vi "KeyDown.vi"(6 "PlatMods":T9, 7 "Type":T1, 8 "error in (no error)":errorcluster, 9 "VKey":T10, 10 "Char":i16, 11 "Data in":T2={"Class"={"Ants"=refnum, "Layer"=refnum, "Templates"=refnum, "Icon"=refnum, "Glyph"=refnum, "Settings"=refnum, "Tools"=refnum}, "Ref"={"Add Layer"=refnum, "Remove Layer"=refnum, "Line Text"=[], "Body Text Spec"=refnum, "DNL_Font"=refnum, "glyph path str"=refnum, "templates path str"=refnum, "Arrow Up"=refnum, "Arrow Down"=refnum, "IE VI Ref"=refnum, "Glyphs tree"=refnum, "Templates tree"=refnum, "Layer Icon Text"=refnum, "Layer Template"=refnum, "Clipboard"=refnum, "BW icon in"=refnum, "Color icon in"=refnum, "Layer Clust"=refnum, "Body Text"=refnum, "DNL_Framework Templates"=refnum, "Search Templates"=refnum, "TextMarker"=refnum, "Tab Control"=refnum, "Search Glyphs"=refnum, "Line Color"=refnum, "DNL_Glyphs []"=refnum, "Fill Color"=refnum, "Tools"=refnum, "Glyphs tree"=refnum, "Icon"=refnum, "Preview"=refnum, "Ants"=refnum, "Terminals"=refnum, "menu reference"=refnum, "LayerNames"=[], "GlyphLoadAnimation"=refnum, "TemplateLoadAnimation"=refnum, "refreshGlyphs"=refnum, "refreshTemplates"=refnum}, "Support"={"AntsRect"={"left"=0, "top"=0, "right"=0, "bottom"=0}, "Mouse Move Coords"={"Horizontal"=0, "Vertical"=0}, "Mouse Down Coords"={"Horizontal"=0, "Vertical"=0}, "Temp Coord"={"Horizontal"=0, "Vertical"=0}, "Action"=enum."Default", "Edge Color"=4914962, "Fill Color"=16860, "Mouse Down?"=FALSE, "Draft Mode?"=FALSE, "Temp Icon"=bytes[3102], "CTRL Pressed"=FALSE, "Move Selection?"=FALSE, "AntsRect Orig"={"left"=0, "top"=0, "right"=0, "bottom"=0}, "Text"="", "TM Set?"=FALSE, "Mouse inside icon?"=FALSE, "Tool (old value)"=0, "Pencil Move Color"=0, "Swap Colors?"=FALSE, "Shift pressed?"=FALSE}}) -> (0 "error out":errorcluster, 1 "Discard?":bool, 3 "Data out":T2={"Class"={"Ants"=refnum, "Layer"=refnum, "Templates"=refnum, "Icon"=refnum, "Glyph"=refnum, "Settings"=refnum, "Tools"=refnum}, "Ref"={"Add Layer"=refnum, "Remove Layer"=refnum, "Line Text"=[], "Body Text Spec"=refnum, "DNL_Font"=refnum, "glyph path str"=refnum, "templates path str"=refnum, "Arrow Up"=refnum, "Arrow Down"=refnum, "IE VI Ref"=refnum, "Glyphs tree"=refnum, "Templates tree"=refnum, "Layer Icon Text"=refnum, "Layer Template"=refnum, "Clipboard"=refnum, "BW icon in"=refnum, "Color icon in"=refnum, "Layer Clust"=refnum, "Body Text"=refnum, "DNL_Framework Templates"=refnum, "Search Templates"=refnum, "TextMarker"=refnum, "Tab Control"=refnum, "Search Glyphs"=refnum, "Line Color"=refnum, "DNL_Glyphs []"=refnum, "Fill Color"=refnum, "Tools"=refnum, "Glyphs tree"=refnum, "Icon"=refnum, "Preview"=refnum, "Ants"=refnum, "Terminals"=refnum, "menu reference"=refnum, "LayerNames"=[], "GlyphLoadAnimation"=refnum, "TemplateLoadAnimation"=refnum, "refreshGlyphs"=refnum, "refreshTemplates"=refnum}, "Support"={"AntsRect"={"left"=0, "top"=0, "right"=0, "bottom"=0}, "Mouse Move Coords"={"Horizontal"=0, "Vertical"=0}, "Mouse Down Coords"={"Horizontal"=0, "Vertical"=0}, "Temp Coord"={"Horizontal"=0, "Vertical"=0}, "Action"=enum."Default", "Edge Color"=4914962, "Fill Color"=16860, "Mouse Down?"=FALSE, "Draft Mode?"=FALSE, "Temp Icon"=bytes[3102], "CTRL Pressed"=FALSE, "Move Selection?"=FALSE, "AntsRect Orig"={"left"=0, "top"=0, "right"=0, "bottom"=0}, "Text"="", "TM Set?"=FALSE, "Mouse inside icon?"=FALSE, "Tool (old value)"=0, "Pencil Move Color"=0, "Swap Colors?"=FALSE, "Shift pressed?"=FALSE}})   [LabVIEW 2021]
uses:
  <vilib>/event_ctls.llb/eventvkey.ctl
  Controls/IE Data.ctl
  Class/Ants/Ants.lvclass
  Class/FakedArray/FakedArray.lvclass
  vi.lib/LabVIEW Icon API/lv_icon/Classes/Icon/Icon.lvclass
  Class/Icon Library/Glyph.lvclass
  Class/Settings/Settings.lvclass
  Class/Tools/Tools Paint.lvclass
  Controls/IE Classes.ctl
  Controls/References Cluster.ctl
  Controls/SupportClass.ctl
  <vilib>/Utility/miscctls.llb/LVPoint32TypeDef.ctl
  Controls/SupportClass_Action.ctl
  vi.lib/LabVIEW Icon API/lv_icon/Controls/IEColor.ctl
  <vilib>/event_ctls.llb/lveventtype.ctl
  vi.lib/LabVIEW Icon API/lv_icon/lv_icon.lvlib
panel:
  in  "Layer name":string="Clipboard"
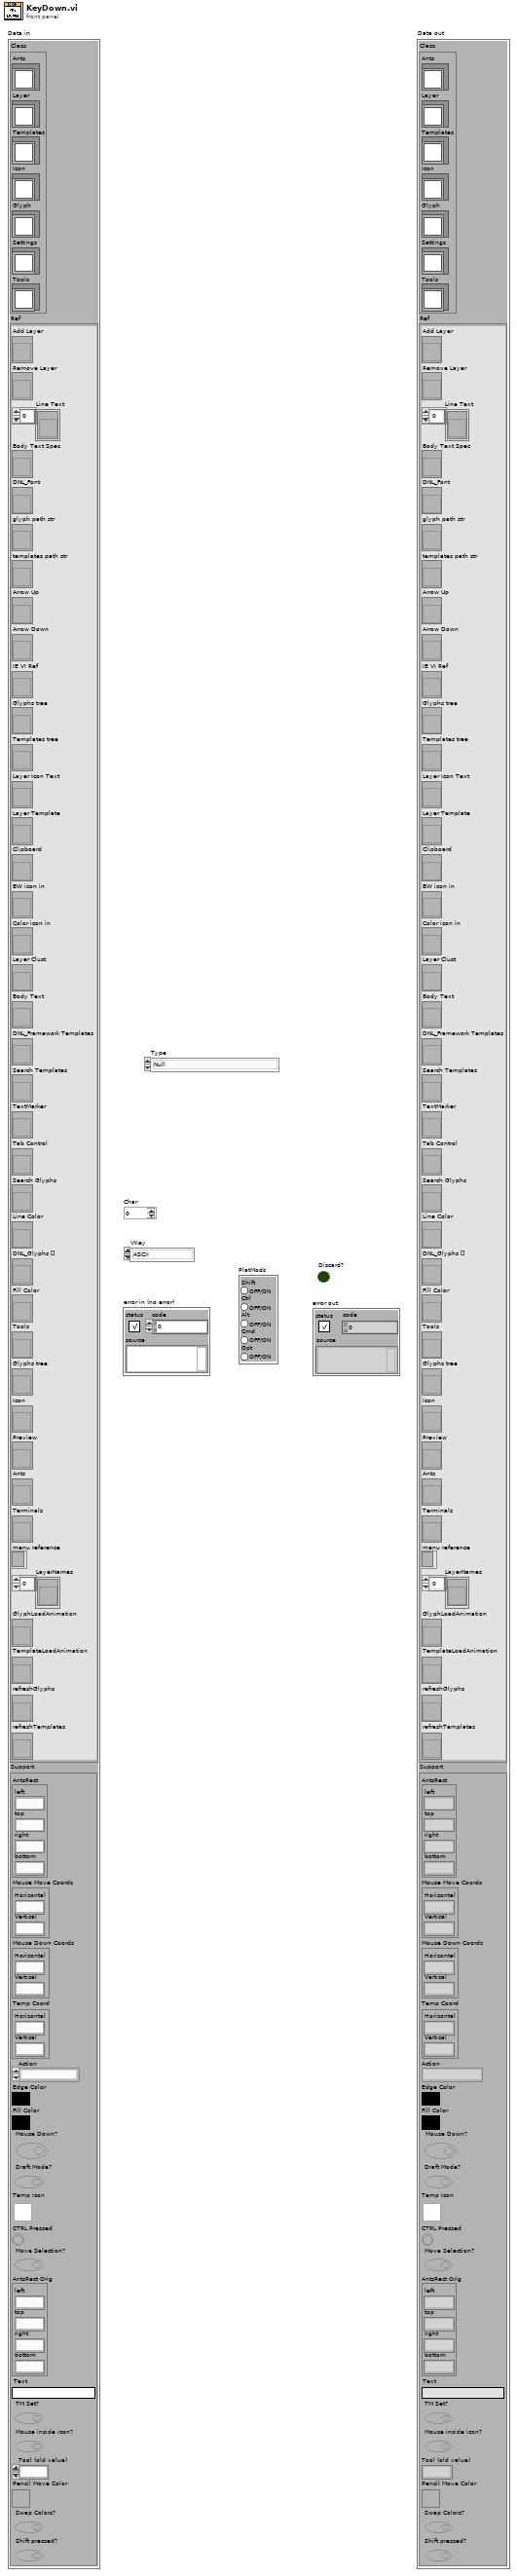
[diagram p1: front panel]
types:
  T1 = typedef "lveventtype.ctl" = enum32{"Null", "Timeout", "Annotation Menu Selection", "Annotation Menu Selection?", "App Instance Close", "App Instance Close?", "Autoscale Range Change", "Bookmark Info Change", "Cell Edit", "Cell Edit?", "Cursor Grab", "Cursor Grab?", "Cursor Menu Selection", "Cursor Menu Selection?", "Cursor Move", "Cursor Release", "Data Change", "Direction Change", "Display State Change", "Drag Ended", "Drag Enter", "Drag Leave", "Drag Over", "Drag Source Update", "Drag Starting", "Drag Starting?", "Drop", "Exec State Change", "Key Down", "Key Down?", "Key Repeat", "Key Repeat?", "Key Up", "Listbox Double Click", "Menu Activation?", "Menu Selection (App)", "Menu Selection? (App)", "Menu Selection (User)", "Mouse Down", "Mouse Down?", "Mouse Enter", "Mouse Leave", "Mouse Move", "Mouse Up", "Mouse Wheel", "NI Security User Change (App)", "Pane Size", "Panel Close", "Panel Close?", "Panel Resize", "Plot Attribute Change", "Scale Range Change", "Shortcut Menu Activation?", "Shortcut Menu Selection (App)", "Shortcut Menu Selection? (App)", "Shortcut Menu Selection (User)", "Tree Double Click", "Tree Drag", "Tree Drag?", "Tree Drop", "Tree Drop?", "Tree Item Close", "Tree Item Close?", "Tree Item Open", "Tree Item Open?", "User Event", "Value Change"}
  T2 = typedef "IE Data.ctl" = cluster{"Class":T3, "Ref":T4, "Support":T5}
  T3 = typedef "IE Classes.ctl" = cluster{"Ants":refnum<class "Ants.lvclass">, "Layer":refnum<class "FakedArray.lvclass">, "Templates":refnum<class "FakedArray.lvclass">, "Icon":refnum<class "Icon.lvclass">, "Glyph":refnum<class "Glyph.lvclass">, "Settings":refnum<class "Settings.lvclass">, "Tools":refnum<class "Tools Paint.lvclass">}
  T4 = typedef "References Cluster.ctl" = cluster{"Add Layer":refnum<vi>, "Remove Layer":refnum<vi>, "Line Text":refnum<vi>[], "Body Text Spec":refnum<vi>, "DNL_Font":refnum<vi>, "glyph path str":refnum<vi>, "templates path str":refnum<vi>, "Arrow Up":refnum<vi>, "Arrow Down":refnum<vi>, "IE VI Ref":refnum<vi>, "Glyphs tree":refnum<vi>, "Templates tree":refnum<vi>, "Layer Icon Text":refnum<vi>, "Layer Template":refnum<vi>, "Clipboard":refnum<vi>, "BW icon in":refnum<vi>, "Color icon in":refnum<vi>, "Layer Clust":refnum<vi>, "Body Text":refnum<vi>, "DNL_Framework Templates":refnum<vi>, "Search Templates":refnum<vi>, "TextMarker":refnum<vi>, "Tab Control":refnum<vi>, "Search Glyphs":refnum<vi>, "Line Color":refnum<vi>, "DNL_Glyphs []":refnum<vi>, "Fill Color":refnum<vi>, "Tools":refnum<vi>, "Glyphs tree":refnum<vi>, "Icon":refnum<vi>, "Preview":refnum<vi>, "Ants":refnum<vi>, "Terminals":refnum<vi>, "menu reference":refnum<k9>, "LayerNames":refnum<vi>[], "GlyphLoadAnimation":refnum<vi>, "TemplateLoadAnimation":refnum<vi>, "refreshGlyphs":refnum<vi>, "refreshTemplates":refnum<vi>}
  T5 = typedef "SupportClass.ctl" = cluster{"AntsRect":cluster{"left":i16, "top":i16, "right":i16, "bottom":i16}, "Mouse Move Coords":T6, "Mouse Down Coords":T6, "Temp Coord":T6, "Action":T7, "Edge Color":T8, "Fill Color":T8, "Mouse Down?":bool, "Draft Mode?":bool, "Temp Icon":picture, "CTRL Pressed":bool, "Move Selection?":bool, "AntsRect Orig":cluster{"left":i16, "top":i16, "right":i16, "bottom":i16}, "Text":string, "TM Set?":bool, "Mouse inside icon?":bool, "Tool (old value)":u32, "Pencil Move Color":u32, "Swap Colors?":bool, "Shift pressed?":bool}
  T6 = typedef "LVPoint32TypeDef.ctl" = cluster{"Horizontal":i32, "Vertical":i32}
  T7 = typedef "SupportClass_Action.ctl" = enum16{"Default", "Move Selection", "Glyph Library", "Tool"}
  T8 = typedef "IEColor.ctl" = u32
  T9 = cluster{"Shift":bool, "Ctrl":bool, "Alt":bool, "Cmd":bool, "Opt":bool}
  T10 = typedef "eventvkey.ctl" = enum16{"ASCII", "Enter", "Return", "Shift", "Ctrl", "Alt", "Cmd", "Opt", "Caps", "NumLock", "Clear", "Break", "Up", "Down", "Left", "Right", "Insert", "Delete", "Home", "End", "PageUp", "PageDown", "Escape", "Help", "Pause", "ScrollLock", "F1", "F2", "F3", "F4", "F5", "F6", "F7", "F8", "F9", "F10", "F11", "F12", "F13", "F14", "F15", "F16", "F17", "F18", "F19", "F20", "F21", "F22", "F23", "F24", "Play", "VolumeUp", "VolumeDown", "Mute", "Two Byte Char"}
  T11 = cluster{"left":i16, "top":i16, "right":i16, "bottom":i16}
  T12 = enum32{"Pencil", "Line", "Dropper", "Fill", "Rectangle", "Filled Rectangle", "Ellipse", "Filled Ellipse", "Eraser", "Text", "Select", "Move"}
  T13 = typedef "Graphic.ctl" = cluster{"Rectangle":cluster{"left":i16, "top":i16, "right":i16, "bottom":i16}, "Path":path, "Image":picture, "Filter":string, "FileName":string}
  T14 = cluster{"left":i16, "top":i16, "bottom":i16, "right":i16}
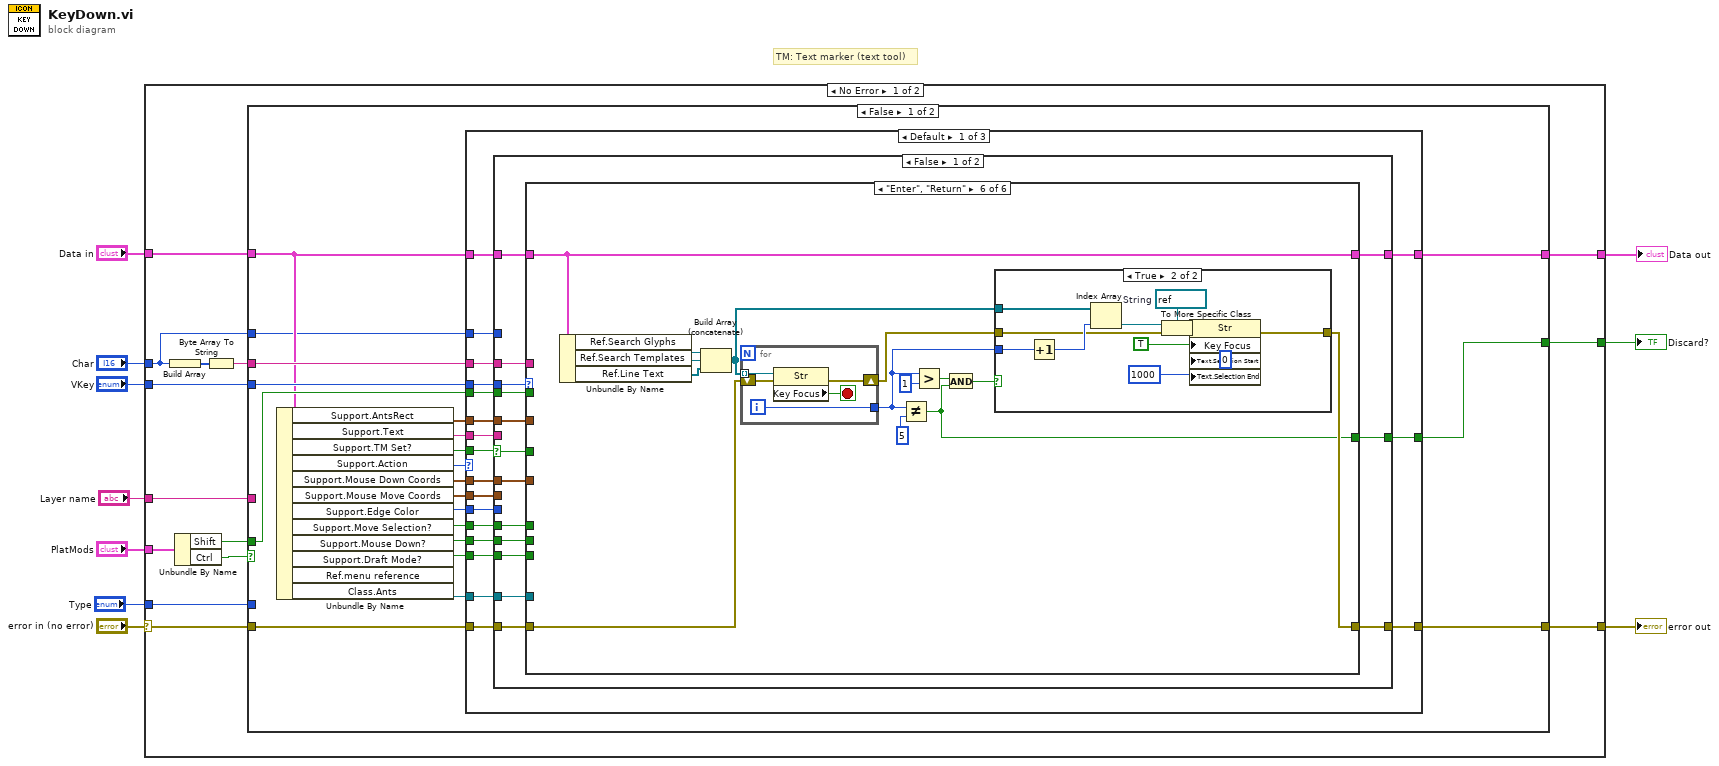
[diagram p0: block diagram]
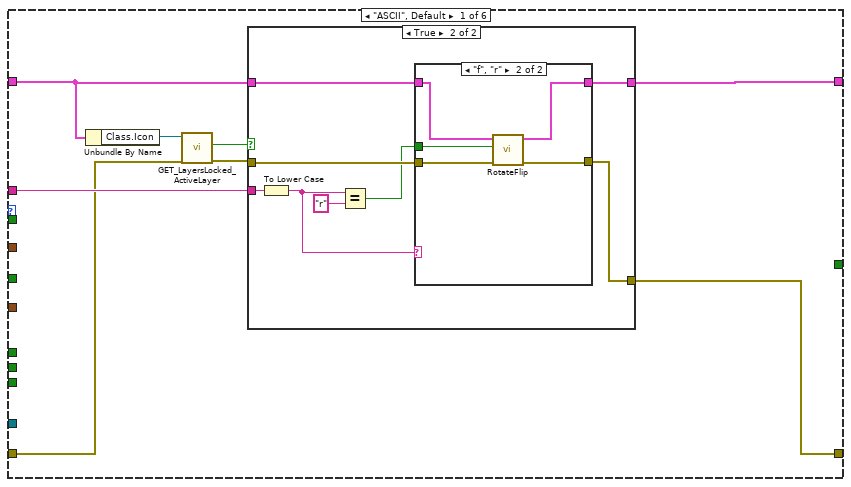
[diagram p2: hidden frame]
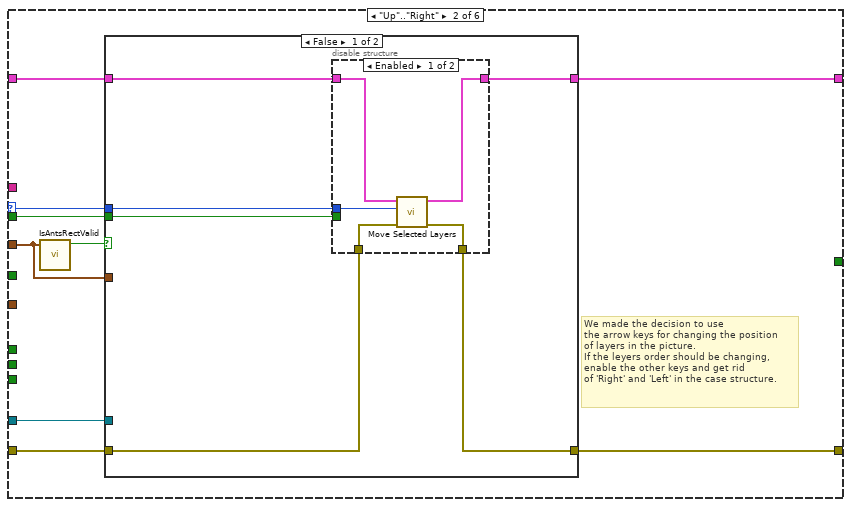
[diagram p5: hidden frame]
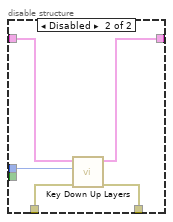
[diagram p6: hidden frame]
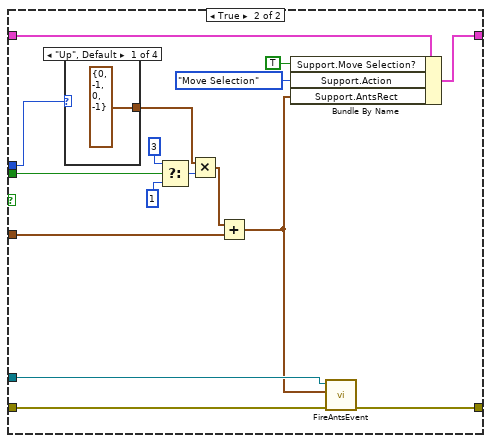
[diagram p7: hidden frame]
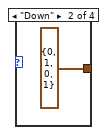
[diagram p8: hidden frame]
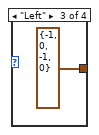
[diagram p9: hidden frame]
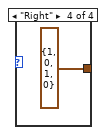
[diagram p10: hidden frame]
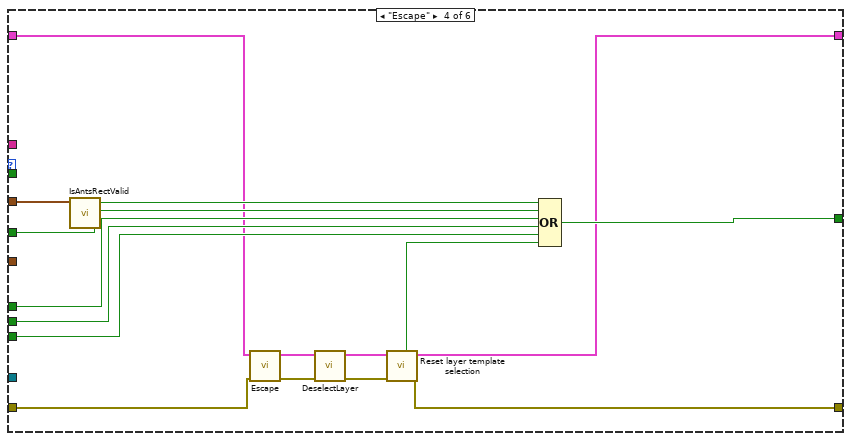
[diagram p12: hidden frame]
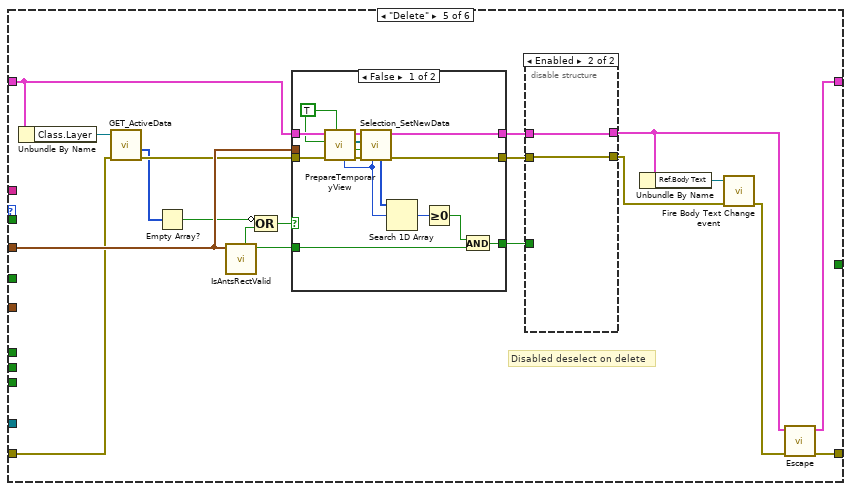
[diagram p13: hidden frame]
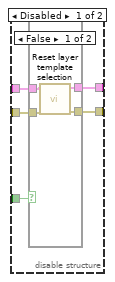
[diagram p14: hidden frame]
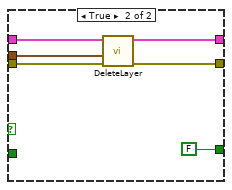
[diagram p16: hidden frame]
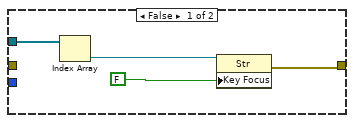
[diagram p17: hidden frame]
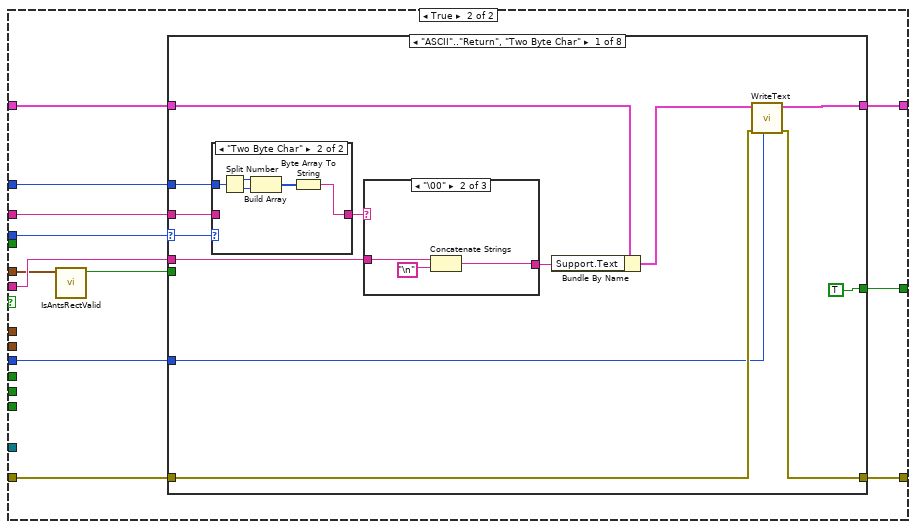
[diagram p18: hidden frame]
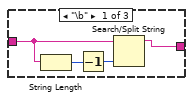
[diagram p20: hidden frame]
diagram:
  # "TM: Text marker (text tool)"
  n1 = case shown="No Error" "error in (no error)" {
    selector: "error in (no error)" -> [w17 w754]
    tunnel: [w21 w754] -> w9
    tunnel: "VKey" -> [w24 _]
    tunnel: "Char" -> [w12 _]
    tunnel: "PlatMods" -> [w20 _]
    tunnel: [w18 _] -> w5
    tunnel: "Data in" -> [w15 w753]
    tunnel: [w14 w753] -> w3
    tunnel: "Type" -> [w13 _]
    tunnel: "Layer name" -> [w11 _]
    frame No Error {
      n2 = Build Array(w12) -> (w23:i16[])
      n3 = Unbundle By Name(w20) -> ("Shift"=w16:bool, "Ctrl"=w19:bool)
      n4 = Byte Array To String(unsigned byte array=w23) -> (string=w22:string)
      n5 = case shown="False" w19 {
        selector: w19 -> [_ w541]
        tunnel: w24 -> [w44 _]
        tunnel: w22 -> [w43 w539]
        tunnel: [w28 w551] -> w21
        tunnel: [w32 w538] -> w18
        tunnel: w17 -> [w30 w554]
        tunnel: w16 -> [w31 w542]
        tunnel: w15 -> [w29 w553]
        tunnel: [w26 w552] -> w14
        tunnel: w13 -> [_ w546]
        tunnel: w12 -> [w25 _]
        tunnel: w11 -> [_ w536]
        frame False {
          n6 = Unbundle By Name(w29) -> ("Support.AntsRect"=w37:T11, "Support.Text"=w40:string, "Support.TM Set?"=w41:bool, "Support.Action"=w42:T7, "Support.Mouse Down Coords"=w39:T6, "Support.Mouse Move Coords"=w36:T6, "Support.Edge Color"=w38:T8, "Support.Move Selection?"=w35:bool, "Support.Mouse Down?"=w34:bool, "Support.Draft Mode?"=w33:bool, "Class.Ants"=w27:refnum<class "Ants.lvclass">)  [unwired: 1 out]
          n7 = case shown="Default" w42 {
            tunnel: w44 -> [w63 w363 w430]
            tunnel: w43 -> [w58 w362 _]
            tunnel: w30 -> [w61 w361 w432]
            tunnel: [w62 w360 w431] -> w28
            tunnel: w41 -> [w60 w358 w428]
            tunnel: w40 -> [w59 _ _]
            tunnel: w39 -> [w57 _ _]
            tunnel: w38 -> [w56 _ _]
            tunnel: w37 -> [w55 w359 w429]
            tunnel: w36 -> [w54 w351 _]
            tunnel: w35 -> [w53 w357 w427]
            tunnel: w34 -> [w52 w356 w426]
            tunnel: w33 -> [w51 w355 w425]
            tunnel: [w50 w354 w424] -> w32
            tunnel: w31 -> [w49 _ w420]
            tunnel: w29 -> [w48 w353 w423]
            tunnel: [w47 w352 w422] -> w26
            tunnel: w27 -> [w45 _ w421]
            tunnel: w25 -> [w46 _ _]
            frame Default {
              n8 = case shown="False" w60 {
                selector: w60 -> [w69 _]
                tunnel: w63 -> [w77 w265]
                tunnel: [w76 w264] -> w62
                tunnel: w61 -> [w78 w263]
                tunnel: w59 -> [_ w262]
                tunnel: w58 -> [w75 w261]
                tunnel: w57 -> [w73 _]
                tunnel: w56 -> [_ w258]
                tunnel: w55 -> [w74 w260]
                tunnel: w54 -> [_ _]
                tunnel: w53 -> [w72 _]
                tunnel: w52 -> [w71 _]
                tunnel: w51 -> [w70 _]
                tunnel: [w68 w257] -> w50
                tunnel: w49 -> [w67 _]
                tunnel: w48 -> [w66 w256]
                tunnel: [w65 w255] -> w47
                tunnel: w46 -> [_ w254]
                tunnel: w45 -> [w64 _]
                frame False {
                  n9 = case shown="\"Enter\", \"Return\"" w77 {
                    selector: w77 -> [_ w110 _ _ _ _]
                    tunnel: w78 -> [w82 w112 w150 w166 w174 w232]
                    tunnel: [w85 w111 w150 w163 w185 w229] -> w76
                    tunnel: w75 -> [w86 _ _ _ _ _]
                    tunnel: w74 -> [_ w105 _ w161 w178 _]
                    tunnel: w73 -> [_ _ _ _ _ _]
                    tunnel: w72 -> [_ _ _ w159 _ _]
                    tunnel: w71 -> [_ _ _ w158 _ _]
                    tunnel: w70 -> [_ _ _ w157 _ _]
                    tunnel: w69 -> [_ _ _ w160 _ _]
                    tunnel: [_ _ _ w156 _ w221] -> w68
                    tunnel: w67 -> [_ w109 _ _ _ _]
                    tunnel: w66 -> [w84 w108 w149 w154 w175 w233]
                    tunnel: [w83 w107 w149 w151 w184 w233] -> w65
                    tunnel: w64 -> [_ w104 _ _ _ _]
                    frame "ASCII", Default {
                      n10 = Unbundle By Name(w84) -> ("Class.Icon"=w80:refnum<class "Icon.lvclass">)
                      n11 = call-dynamic "GET_LayersLocked_ActiveLayer.vi"("error in (no error)"=w82, "Icon.lvclass in"=w80) -> ("error out"=w81:errorcluster, "Layers Locked?"=w79:bool)  [unwired: 8 out]
                      n12 = case shown="True" w79 {
                        tunnel: w86 -> [_ w93]
                        tunnel: w81 -> [w88 w96]
                        tunnel: [w88 w95] -> w85
                        tunnel: w84 -> [w87 w90]
                        tunnel: [w87 w89] -> w83
                        frame False {
                        }
                        frame True {
                          n13 = To Lower Case(string=w93) -> (all lower case string=w91:string)
                          n14 = Equal?(x=w91, y="r") -> (x = y?=w92:bool)
                          n15 = case shown="\"f\", \"r\"" w91 {
                            tunnel: w96 -> [w98 w103]
                            tunnel: [w98 w101] -> w95
                            tunnel: w92 -> [_ w102]
                            tunnel: w90 -> [w97 w100]
                            tunnel: [w97 w99] -> w89
                            frame Default {
                            }
                            frame "f", "r" {
                              n16 = call "RotateFlip.vi"("error in"=w103, "Rotate"=w102, "Data in"=w100) -> ("error out"=w101:errorcluster, "Data out"=w99:T2)  [unwired: 3 in, 4 out]
                            }
                          }
                        }
                      }
                    }
                    frame "Up".."Right" {
                      # "We made the decision to use\nthe arrow keys for changing the position\nof layers in the picture.\nIf the leyers order should be changing,\nenable the other keys and get rid\nof 'Right' and 'Left' in the case structure."
                      n17 = call "IsAntsRectValid.vi"("AntsRect"=w105) -> ("Valid?"=w106:bool)  [unwired: 10 out]
                      n18 = case shown="False" w106 {
                        tunnel: w112 -> [w118 w132]
                        tunnel: [w117 w131] -> w111
                        tunnel: w110 -> [w116 w135]
                        tunnel: w109 -> [w115 w134]
                        tunnel: w108 -> [w114 w144]
                        tunnel: [w113 w142] -> w107
                        tunnel: w105 -> [_ w133]
                        tunnel: w104 -> [_ w130]
                        frame False {
                          n19 = disable-structure shown="Enabled" {
                            disable-tunnel: w118 -> [w121 w126]
                            disable-tunnel: [w120 w125] -> w117
                            disable-tunnel: w116 -> [w119 w124]
                            disable-tunnel: w115 -> [_ _]
                            disable-tunnel: w114 -> [w123 w128]
                            disable-tunnel: [w122 w127] -> w113
                            frame Enabled {
                              n20 = call "Move Selected Layers.vi"("error in"=w121, "VKey"=w119, "Data in"=w123) -> ("error out"=w120:errorcluster, "Data out"=w122:T2)  [unwired: 1 in, 6 out]
                            }
                            frame Disabled {
                              n21 = call "Key Down Up Layers.vi"("error in"=w126, "VKey"=w124, "Data in"=w128) -> ("error out"=w125:errorcluster, "Data out"=w127:T2)  [unwired: 1 in, 6 out]
                            }
                          }
                        }
                        frame True {
                          n22 = case shown="\"Up\", Default" w135 {
                            tunnel: [T11 {"left"=0, "top"=-1, "right"=0, "bottom"=-1} ("y") T11 {"left"=0, "top"=1, "right"=0, "bottom"=1} ("y") T11 {"left"=-1, "top"=0, "right"=-1, "bottom"=0} ("y") T11 {"left"=1, "top"=0, "right"=1, "bottom"=0} ("y")] -> w140
                            frame "Up", Default {
                            }
                            frame "Down" {
                            }
                            frame "Left" {
                            }
                            frame "Right" {
                            }
                          }
                          n23 = Select(t=i16 3 ("left"), s=w134, f=i16 1 ("left")) -> (s? t:f=w137:i16)
                          n24 = Multiply(x=w140, y=w137) -> (x*y=w136:T11)
                          n25 = Add(x=w136, y=w133) -> (x+y=w129:T11)
                          n26 = Bundle By Name(cluster=w144, "Support.Move Selection?"=TRUE, "Support.Action"=SupportClass_Action."Move Selection", "Support.AntsRect"=w129) -> (w142:T2)
                          n27 = call "FireAntsEvent.vi"("error in (no error)"=w132, "Rectangle (default: deselect)"=w129, "Ants in"=w130) -> ("error out"=w131:errorcluster)  [unwired: 1 in, 7 out]
                        }
                      }
                    }
                    frame "Shift" {
                    }
                    frame "Escape" {
                      n28 = call "IsAntsRectValid.vi"("AntsRect"=w161) -> ("Valid?"=w162:bool)  [unwired: 10 out]
                      n29 = call "Escape.vi"("error in"=w166, "Data in"=w154) -> ("error out"=w165:errorcluster, "Data out"=w153:T2)  [unwired: 8 out]
                      n30 = call "DeselectLayer.vi"("error in (no error)"=w165, "Data in"=w153) -> ("error out"=w164:errorcluster, "Data out"=w152:T2)  [unwired: 8 out]
                      n31 = call "Reset layer template selection.vi"("error in (no error)"=w164, "Data in"=w152) -> ("error out"=w163:errorcluster, "Data out"=w151:T2, "Layers selected?"=w155:bool)  [unwired: 1 in, 6 out]
                      n32 = Compound Arithmetic op=OR(w162, w160, w159, w158, w157, w155) -> (w156:bool)
                    }
                    frame "Delete" {
                      # "Disabled deselect on delete"
                      n33 = Unbundle By Name(w175) -> ("Class.Layer"=w176:refnum<class "FakedArray.lvclass">)
                      n34 = call-dynamic "GET_ActiveData.vi"("error in (no error)"=w174, "FakedArray in"=w176) -> ("error out"=w173:errorcluster, "Active Data []"=w172:i32[])  [unwired: 4 in, 4 out]
                      n35 = Empty Array?(array=w172) -> (empty?=w170:bool)
                      n36 = call "IsAntsRectValid.vi"("AntsRect"=w178) -> ("Valid?"=w183:bool, "Max. Rect size?"=w171:bool)  [unwired: 9 out]
                      n37 = Compound Arithmetic op=OR(invert w170, w171) -> (w169:bool)
                      n38 = case shown="False" w169 {
                        tunnel: w183 -> [w213 _]
                        tunnel: w175 -> [w212 w219]
                        tunnel: [w211 w217] -> w182
                        tunnel: [w210 w218] -> w181
                        tunnel: w173 -> [w200 w216]
                        tunnel: w178 -> [_ w215]
                        tunnel: [w199 FALSE] -> w179
                        frame False {
                          w209 = TRUE ("Delete Selected Area?")
                          n39 = call "PrepareTemporaryView.vi"("Delete Selected Area?"=w209, "error in (no error)"=w200, "Valid Selection?"=w209, "Data in"=w212) -> ("error out"=w206:errorcluster, "Highlighted?"=w207:bool, "All Layers out"=w208:refnum<class "Layer.lvclass">[], "Data out"=w201:T2, "#Active Layer"=w204:i32)  [unwired: 1 in, 2 out]
                          n40 = call "Selection_SetNewData.vi"("#Active Layer"=w204, "error in"=w206, "Highlighted?"=w207, "All Layers In"=w208, "Data in"=w201) -> ("error out"=w211:errorcluster, "Data out"=w210:T2, "Remaining Indices"=w205:i32[])  [unwired: 1 in, 2 out]
                          n41 = Search 1D Array(1D array=w205, element=w204) -> (index of element=w203:i32)  [unwired: 1 out]
                          n42 = Greater Or Equal To 0?(x=w203) -> (x >= 0?=w202:bool)
                          n43 = And(x=w202, y=w213) -> (x .and. y?=w199:bool)
                        }
                        frame True {
                          n44 = call "DeleteLayer.vi"("error in"=w216, "AntsRect"=w215, "Data in"=w219) -> ("error out"=w217:errorcluster, "Data out"=w218:T2)  [unwired: 5 out]
                        }
                      }
                      n45 = disable-structure shown="Enabled" {
                        disable-tunnel: w182 -> [w190 w198]
                        disable-tunnel: w181 -> [w189 w197]
                        disable-tunnel: [w188 w197] -> w168
                        disable-tunnel: [w187 w198] -> w180
                        disable-tunnel: w179 -> [w186 _]
                        frame Disabled {
                          n46 = case shown="False" w186 {
                            tunnel: w190 -> [w194 w195]
                            tunnel: w189 -> [w193 w196]
                            tunnel: [w192 w196] -> w188
                            tunnel: [w191 w195] -> w187
                            frame False {
                              n47 = call "Reset layer template selection.vi"("error in (no error)"=w194, "Data in"=w193) -> ("error out"=w191:errorcluster, "Data out"=w192:T2)  [unwired: 1 in, 7 out]
                            }
                            frame True {
                            }
                          }
                        }
                        frame Enabled {
                        }
                      }
                      n48 = Unbundle By Name(w168) -> ("Ref.Body Text"=w167:refnum<vi>)
                      n49 = call "Fire Body Text Change event.vi"("error in"=w180, "Ref.Body Text"=w167) -> ("error out"=w177:errorcluster)  [unwired: 2 in, 7 out]
                      n50 = call "Escape.vi"("error in"=w177, "Data in"=w168) -> ("error out"=w185:errorcluster, "Data out"=w184:T2)  [unwired: 8 out]
                    }
                    frame "Enter", "Return" {
                      n51 = Unbundle By Name(w233) -> ("Ref.Search Glyphs"=w225:refnum<vi>, "Ref.Search Templates"=w226:refnum<vi>, "Ref.Line Text"=w228:refnum<vi>[])
                      n52 = Build Array (concatenate)(w225, w226, w228) -> (w227:refnum<vi>[])
                      n53 = for {
                        tunnel: w227 -> [w253] mode=indexing
                        shift-right: [w252] -> w230
                        shift-left: w232 -> [w251]
                        tunnel: [w250] -> w224
                        i -> [w250]
                        stop <- w249 stop-if-true
                        n54 = property class="Str"(reference=w253, error in=w251) -> (error out=w252:errorcluster, "Key Focus"=w249:bool)  [unwired: 1 out]
                      }
                      n55 = Not Equal?(x=w224, y=5) -> (x != y?=w221:bool)
                      n56 = Greater?(x=w224, y=1) -> (0:w222:bool)
                      n57 = And(x=w222, y=w221) -> (x .and. y?=w220:bool)
                      n58 = case shown="True" w220 {
                        tunnel: w224 -> [_ w247]
                        tunnel: w227 -> [w237 w248]
                        tunnel: w230 -> [_ w244]
                        tunnel: [w234 w242] -> w229
                        frame False {
                          n59 = Index Array(array=w237) -> (element=w236:refnum<vi>)  [unwired: 1 in]
                          n60 = property class="Str"(reference=w236, "Key Focus"=FALSE) -> (error out=w234:errorcluster)  [unwired: 1 in, 1 out]
                        }
                        frame True {
                          w238 = refnum<vi> refnum  # String
                          n61 = Increment(x=w247) -> (x+1=w246:i32)
                          n62 = Index Array(array=w248, index=w246) -> (element=w245:refnum<vi>)
                          n63 = To More Specific Class(target class=w238, reference=w245) -> (specific class reference=w239:refnum<vi>)  [unwired: 1 in, 1 out]
                          n64 = property class="Str"(reference=w239, error in=w244, "Key Focus"=TRUE, "Text.Selection Start"=u32 0 ("Text.Selection:Start"), "Text.Selection End"=u32 1000 ("Text.Selection:End")) -> (error out=w242:errorcluster)  [unwired: 1 out]
                        }
                      }
                    }
                  }
                }
                frame True {
                  n65 = call "IsAntsRectValid.vi"("AntsRect"=w260) -> ("Valid?"=w259:bool)  [unwired: 10 out]
                  n66 = case shown="\"ASCII\"..\"Return\", \"Two Byte Char\"" w265 {
                    selector: w265 -> [w269 _ _ _ _ _ _ _]
                    tunnel: [w276 w298 w301 w305 w330 w336 w342 w348] -> w264
                    tunnel: w263 -> [w277 w299 w301 w306 w331 w337 w343 w349]
                    tunnel: w262 -> [w278 _ _ w307 _ _ _ _]
                    tunnel: w261 -> [w267 _ _ _ _ _ _ _]
                    tunnel: w258 -> [w275 _ _ _ w332 w338 w344 w350]
                    tunnel: w259 -> [_ _ _ w304 _ _ _ _]
                    tunnel: [TRUE TRUE _ _ _ _ _ _] -> w257
                    tunnel: w256 -> [w270 w296 w300 w303 w329 w334 w341 w347]
                    tunnel: [w273 w295 w300 w302 w327 w333 w340 w345] -> w255
                    tunnel: w254 -> [w266 _ _ _ _ _ _ _]
                    frame "ASCII".."Return", "Two Byte Char" {
                      n67 = case shown="\"Two Byte Char\"" w269 {
                        tunnel: [w279 w280] -> w268
                        tunnel: w267 -> [w279 _]
                        tunnel: w266 -> [_ w284]
                        frame "ASCII", Default {
                        }
                        frame "Two Byte Char" {
                          n68 = Split Number(x=w284) -> (hi(x)=w282:u8, lo(x)=w283:u8)
                          n69 = Build Array(w282, w283) -> (w281:u8[])
                          n70 = Byte Array To String(unsigned byte array=w281) -> (string=w280:string)
                        }
                      }
                      n71 = case shown="\"\\00\"" w268 {
                        selector: w268 -> [_ _ w292]
                        tunnel: w278 -> [w286 w291 w294]
                        tunnel: [w285 w290 w293] -> w272
                        frame "\b" {
                          n72 = String Length(string=w286) -> (length=w288:i32)
                          n73 = Decrement(x=w288) -> (x-1=w287:i32)
                          n74 = Search/Split String(string=w286, offset (0)=w287) -> (substring before match=w285:string)  [unwired: 3 out]
                        }
                        frame "\u0000\u0000" {
                          n75 = Concatenate Strings(w291, "\n") -> (w290:string)
                        }
                        frame Default {
                          n76 = Concatenate Strings(w294, w292) -> (w293:string)
                        }
                      }
                      n77 = Bundle By Name(cluster=w270, "Support.Text"=w272) -> (w271:T2)
                      n78 = call "WriteText.vi"("Text Color"=w275, "error in (no error)"=w277, "Data in"=w271) -> ("error out"=w276:errorcluster, "Data out"=w273:T2)  [unwired: 2 in, 5 out]
                    }
                    frame "Escape" {
                      n79 = call "Escape.vi"("error in"=w299, "Data in"=w296) -> ("error out"=w298:errorcluster, "Data out"=w295:T2)  [unwired: 8 out]
                    }
                    frame Default {
                    }
                    frame "Delete" {
                      n80 = case shown="True" w304 {
                        tunnel: w307 -> [_ _]
                        tunnel: w306 -> [w309 w318]
                        tunnel: [w309 w321] -> w305
                        tunnel: w303 -> [w308 w311]
                        tunnel: [w308 w315] -> w302
                        frame False {
                        }
                        frame True {
                          w326 = TRUE ("Delete Selected Area?")
                          n81 = Unbundle By Name(w311) -> ("Ref.Body Text"=w310:refnum<vi>)
                          n82 = call "Fire Body Text Change event.vi"("error in"=w318, "Ref.Body Text"=w310) -> ("error out"=w319:errorcluster)  [unwired: 2 in, 7 out]
                          n83 = call "PrepareTemporaryView.vi"("Delete Selected Area?"=w326, "error in (no error)"=w319, "Valid Selection?"=w326, "Data in"=w311) -> ("error out"=w322:errorcluster, "Highlighted?"=w324:bool, "All Layers out"=w325:refnum<class "Layer.lvclass">[], "Data out"=w317:T2, "#Active Layer"=w323:i32)  [unwired: 1 in, 2 out]
                          n84 = call "Selection_SetNewData.vi"("#Active Layer"=w323, "error in"=w322, "Highlighted?"=w324, "All Layers In"=w325, "Data in"=w317) -> ("error out"=w320:errorcluster, "Data out"=w316:T2)  [unwired: 1 in, 3 out]
                          n85 = call "ViewLayer.vi"("Add to Undo?"=TRUE, "error in (no error)"=w320, "Data in"=w316) -> ("error out"=w314:errorcluster, "Data out"=w313:T2)  [unwired: 2 in, 5 out]
                          n86 = call "Escape.vi"("error in"=w314, "Data in"=w313) -> ("error out"=w321:errorcluster, "Data out"=w315:T2)  [unwired: 8 out]
                        }
                      }
                    }
                    frame "Up" {
                      n87 = call "WriteText.vi"("Text Color"=w332, "error in (no error)"=w331, "Offset"=T6 {"Horizontal"=0, "Vertical"=-1} ("y"), "Data in"=w329) -> ("error out"=w330:errorcluster, "Data out"=w327:T2)  [unwired: 1 in, 5 out]
                    }
                    frame "Down" {
                      n88 = call "WriteText.vi"("Text Color"=w338, "error in (no error)"=w337, "Offset"=T6 {"Horizontal"=0, "Vertical"=1} ("y"), "Data in"=w334) -> ("error out"=w336:errorcluster, "Data out"=w333:T2)  [unwired: 1 in, 5 out]
                    }
                    frame "Left" {
                      n89 = call "WriteText.vi"("Text Color"=w344, "error in (no error)"=w343, "Offset"=T6 {"Horizontal"=-1, "Vertical"=0} ("y"), "Data in"=w341) -> ("error out"=w342:errorcluster, "Data out"=w340:T2)  [unwired: 6 out]
                    }
                    frame "Right" {
                      n90 = call "WriteText.vi"("Text Color"=w350, "error in (no error)"=w349, "Offset"=T6 {"Horizontal"=1, "Vertical"=0} ("y"), "Data in"=w347) -> ("error out"=w348:errorcluster, "Data out"=w345:T2)  [unwired: 6 out]
                    }
                  }
                }
              }
            }
            frame "Glyph Library" {
              n91 = case shown="\"Escape\"" w363 {
                tunnel: w361 -> [w368 w415 w418]
                tunnel: [w367 w414 w418] -> w360
                tunnel: w362 -> [w369 _ _]
                tunnel: w359 -> [_ w412 _]
                tunnel: w358 -> [_ w411 _]
                tunnel: w357 -> [_ w410 _]
                tunnel: w356 -> [_ w409 _]
                tunnel: w355 -> [_ w408 _]
                tunnel: [_ w407 _] -> w354
                tunnel: w353 -> [w366 w406 w417]
                tunnel: [w365 w404 w416] -> w352
                tunnel: w351 -> [w364 _ _]
                frame "ASCII", Default {
                  n92 = case shown="Default" w369 {
                    selector: w369 -> [_ w388]
                    tunnel: w368 -> [w371 w374]
                    tunnel: [w371 w373] -> w367
                    tunnel: w366 -> [w370 w378]
                    tunnel: [w370 w375] -> w365
                    tunnel: w364 -> [_ w372]
                    frame Default {
                    }
                    frame "F", "R", "f", "r" {
                      n93 = Unbundle By Name(w378) -> ("Class.Glyph"=w379:refnum<class "Glyph.lvclass">)
                      n94 = call-dynamic "GET_ActiveGlyph.vi"("error in (no error)"=w374, "Glyph.lvclass in"=w379) -> ("error out"=w391:errorcluster, "Path & Icon"=w393:T13, "Glyph.lvclass out"=w392:refnum<class "Glyph.lvclass">)  [unwired: 7 out]
                      n95 = Unbundle By Name(w393) -> ("Image"=w395:picture, "Rectangle"=w394:T11)
                      n96 = Equal?(x=w388, y="r") -> (x = y?=w385:bool)
                      n97 = Equal?(x=w388, y="R") -> (x = y?=w386:bool)
                      n98 = Or(x=w385, y=w386) -> (x .or. y?=w380:bool)
                      n99 = call "Rotate Flip Image.vi"("Rotate?"=w380, "rect"=w394, "Temp Icon In"=w395) -> ("rect out"=w383:T14, "Temp Icon Out"=w384:picture)  [unwired: 7 out]
                      n100 = case shown="False" w380 {
                        tunnel: w384 -> [w400 w402]
                        tunnel: w383 -> [w399 w401]
                        tunnel: [w398 w402] -> w382
                        tunnel: [w397 w401] -> w381
                        frame False {
                          n101 = call "Rotate Flip Image.vi"("Rotate?"=TRUE, "rect"=w399, "Temp Icon In"=w400) -> ("rect out"=w397:T14, "Temp Icon Out"=w398:picture)  [unwired: 7 out]
                        }
                        frame True {
                        }
                      }
                      n102 = Bundle By Name(cluster=w393, "Image"=w382, "Rectangle"=w381) -> (w390:T13)
                      n103 = call "TemporaryGlyphView.vi"("Mouse Coords Pic"=w372, "Path & Icon"=w390) -> ("icon out"=w376:picture)  [unwired: 9 out]
                      n104 = call-dynamic "SET_ActiveGlyph.vi"("error in (no error)"=w391, "Active Glyph"=w390, "Glyph in"=w392) -> ("error out"=w373:errorcluster, "Glyph out"=w377:refnum<class "Glyph.lvclass">)  [unwired: 7 out]
                      n105 = Bundle By Name(cluster=w378, "Class.Glyph"=w377, "Support.Temp Icon"=w376) -> (w375:T2)
                    }
                  }
                }
                frame "Escape" {
                  n106 = call "IsAntsRectValid.vi"("AntsRect"=w412) -> ("Valid?"=w413:bool)  [unwired: 10 out]
                  n107 = Compound Arithmetic op=OR(w413, w411, w410, w409, w408) -> (w407:bool)
                  n108 = call "Escape.vi"("error in"=w415, "Data in"=w406) -> ("error out"=w403:errorcluster, "Data out"=w405:T2)  [unwired: 8 out]
                  n109 = call "Reset layer template selection.vi"("error in (no error)"=w403, "Data in"=w405) -> ("error out"=w414:errorcluster, "Data out"=w404:T2)  [unwired: 1 in, 7 out]
                }
                frame "Ctrl" {
                  n110 = Bundle By Name(cluster=w417, "Support.CTRL Pressed"=TRUE ("CTRL Pressed")) -> (w416:T2)
                }
              }
            }
            frame "Move Selection" {
              n111 = case shown="\"Up\"..\"Right\"" w430 {
                selector: w430 -> [_ w439 _ _]
                tunnel: w432 -> [w434 w437 w471 w483]
                tunnel: [w434 w436 w464 w492] -> w431
                tunnel: w429 -> [_ w441 w478 w482]
                tunnel: w428 -> [_ _ w476 _]
                tunnel: w427 -> [_ _ w475 _]
                tunnel: w426 -> [_ _ w474 _]
                tunnel: w425 -> [_ _ w473 _]
                tunnel: [_ _ w472 _] -> w424
                tunnel: w423 -> [w433 w443 w468 w484]
                tunnel: [w433 w440 w465 w490] -> w422
                tunnel: w421 -> [_ w435 w470 _]
                tunnel: w420 -> [_ w438 _ _]
                frame "ASCII", Default {
                }
                frame "Up".."Right" {
                  n112 = call "IsAntsRectValid.vi"("AntsRect"=w441) -> ("Valid?"=w442:bool)  [unwired: 10 out]
                  n113 = case shown="True" w442 {
                    tunnel: w443 -> [w445 w459]
                    tunnel: w441 -> [_ w457]
                    tunnel: [w445 w458] -> w440
                    tunnel: w439 -> [_ w450]
                    tunnel: w438 -> [_ w455]
                    tunnel: w437 -> [w444 w449]
                    tunnel: [w444 w448] -> w436
                    tunnel: w435 -> [_ w447]
                    frame False {
                    }
                    frame True {
                      n114 = case shown="\"Up\", Default" w450 {
                        tunnel: [T11 {"left"=0, "top"=-1, "right"=0, "bottom"=-1} ("y") T11 {"left"=0, "top"=1, "right"=0, "bottom"=1} ("y") T11 {"left"=-1, "top"=0, "right"=-1, "bottom"=0} ("y") T11 {"left"=1, "top"=0, "right"=1, "bottom"=0} ("y")] -> w456
                        frame "Up", Default {
                        }
                        frame "Down" {
                        }
                        frame "Left" {
                        }
                        frame "Right" {
                        }
                      }
                      n115 = Select(t=i16 3 ("left"), s=w455, f=i16 1 ("left")) -> (s? t:f=w452:i16)
                      n116 = Multiply(x=w456, y=w452) -> (x*y=w451:T11)
                      n117 = Add(x=w451, y=w457) -> (x+y=w446:T11)
                      n118 = Bundle By Name(cluster=w459, "Support.AntsRect"=w446) -> (w458:T2)
                      n119 = call "FireAntsEvent.vi"("error in (no error)"=w449, "Rectangle (default: deselect)"=w446, "Ants in"=w447) -> ("error out"=w448:errorcluster)  [unwired: 1 in, 7 out]
                    }
                  }
                }
                frame "Escape" {
                  n120 = call "IsAntsRectValid.vi"("AntsRect"=w478) -> ("Valid?"=w477:bool)  [unwired: 10 out]
                  n121 = Compound Arithmetic op=OR(w477, w476, w475, w474, w473) -> (w472:bool)
                  n122 = call "FireAntsEvent.vi"("error in (no error)"=w471, "Ants in"=w470) -> ("error out"=w469:errorcluster)  [unwired: 2 in, 7 out]
                  n123 = call "Reset layer template selection.vi"("error in (no error)"=w469, "Data in"=w468) -> ("error out"=w467:errorcluster, "Data out"=w466:T2)  [unwired: 1 in, 7 out]
                  n124 = call "Escape.vi"("error in"=w467, "Data in"=w466) -> ("error out"=w464:errorcluster, "Data out"=w465:T2)  [unwired: 8 out]
                }
                frame "Delete" {
                  # "Disable deselect on delete"
                  n125 = call "IsAntsRectValid.vi"("AntsRect"=w482) -> ("Valid?"=w491:bool, "Max. Rect size?"=w485:bool)  [unwired: 9 out]
                  n126 = case shown="False" w485 {
                    tunnel: w491 -> [w520 _]
                    tunnel: w484 -> [w519 w524]
                    tunnel: [w518 w532] -> w489
                    tunnel: [w517 w533] -> w488
                    tunnel: w483 -> [w507 w522]
                    tunnel: w482 -> [_ w531]
                    tunnel: [w506 FALSE] -> w481
                    frame False {
                      w516 = TRUE ("Delete Selected Area?")
                      n127 = call "PrepareTemporaryView.vi"("Delete Selected Area?"=w516, "error in (no error)"=w507, "Valid Selection?"=w516, "Data in"=w519) -> ("error out"=w513:errorcluster, "Highlighted?"=w514:bool, "All Layers out"=w515:refnum<class "Layer.lvclass">[], "Data out"=w508:T2, "#Active Layer"=w511:i32)  [unwired: 1 in, 2 out]
                      n128 = call "Selection_SetNewData.vi"("#Active Layer"=w511, "error in"=w513, "Highlighted?"=w514, "All Layers In"=w515, "Data in"=w508) -> ("error out"=w518:errorcluster, "Data out"=w517:T2, "Remaining Indices"=w512:i32[])  [unwired: 1 in, 2 out]
                      n129 = Search 1D Array(1D array=w512, element=w511) -> (index of element=w510:i32)  [unwired: 1 out]
                      n130 = Greater Or Equal To 0?(x=w510) -> (x >= 0?=w509:bool)
                      n131 = And(x=w509, y=w520) -> (x .and. y?=w506:bool)
                    }
                    frame True {
                      n132 = Unbundle By Name(w524) -> ("Class.Icon"=w529:refnum<class "Icon.lvclass">)
                      n133 = call-dynamic "GET_All User Layers.vi"("error in (no error)"=w522, "Icon.lvclass in"=w529) -> ("error out"=w528:errorcluster, "User Layer"=w525:refnum<class "Layer.lvclass">[])  [unwired: 7 in, 1 out]
                      n134 = Array Size(array=w525) -> (size(s)=w526:i32)
                      n135 = for {
                        N: w526 -> [_]
                        tunnel: [w534] -> w527 mode=indexing
                        i -> [w534]
                      }
                      n136 = call "Set active Layer programmatically.vi"("error in"=w528, "Active Layer []"=w527, "Data in"=w524) -> ("error out"=w521:errorcluster, "Data out"=w523:T2)  [unwired: 7 in]
                      n137 = call "DeleteLayer.vi"("error in"=w521, "AntsRect"=w531, "Data in"=w523) -> ("error out"=w532:errorcluster, "Data out"=w533:T2)  [unwired: 5 out]
                    }
                  }
                  n138 = disable-structure shown="Disabled" {
                    disable-tunnel: w489 -> [w497 w504]
                    disable-tunnel: w488 -> [w496 w505]
                    disable-tunnel: [w495 w505] -> w480
                    disable-tunnel: [w494 w504] -> w487
                    disable-tunnel: w481 -> [w493 _]
                    frame Disabled {
                      n139 = case shown="False" w493 {
                        tunnel: w497 -> [w501 w502]
                        tunnel: w496 -> [w500 w503]
                        tunnel: [w499 w503] -> w495
                        tunnel: [w498 w502] -> w494
                        frame False {
                          n140 = call "Reset layer template selection.vi"("error in (no error)"=w501, "Data in"=w500) -> ("error out"=w498:errorcluster, "Data out"=w499:T2)  [unwired: 1 in, 7 out]
                        }
                        frame True {
                        }
                      }
                    }
                    frame Enabled {
                    }
                  }
                  n141 = Unbundle By Name(w480) -> ("Ref.Body Text"=w479:refnum<vi>)
                  n142 = call "Fire Body Text Change event.vi"("error in"=w487, "Ref.Body Text"=w479) -> ("error out"=w486:errorcluster)  [unwired: 2 in, 7 out]
                  n143 = call "Escape.vi"("error in"=w486, "Data in"=w480) -> ("error out"=w492:errorcluster, "Data out"=w490:T2)  [unwired: 8 out]
                }
              }
            }
          }
        }
        frame True {
          n144 = Unbundle By Name(w553) -> ("Support.AntsRect"=w535:T11, "Support.Action"=w540:T7, "Support.Mouse Down?"=w549:bool, "Support.Mouse inside icon?"=w550:bool, "Ref.Tools"=w555:refnum<vi>)
          n145 = Equal?(x=lveventtype."Key Repeat", y=w546) -> (x = y?=w544:bool)
          n146 = Equal?(x=lveventtype."Key Repeat?", y=w546) -> (x = y?=w545:bool)
          n147 = Or(x=w544, y=w545) -> (x .or. y?=w543:bool)
          n148 = case shown="\"Default\", Default" w540 {
            tunnel: w555 -> [_ w629 w723]
            tunnel: w554 -> [w560 w628 w726]
            tunnel: w553 -> [w562 w627 w731]
            tunnel: [w559 w626 w730] -> w552
            tunnel: [w558 w625 w725] -> w551
            tunnel: w550 -> [_ w624 _]
            tunnel: w549 -> [_ w623 _]
            tunnel: w542 -> [_ w622 w728]
            tunnel: w541 -> [_ w621 w724]
            tunnel: w539 -> [w561 w619 w729]
            tunnel: [w557 w618 w727] -> w537
            tunnel: w536 -> [w556 w617 _]
            tunnel: w535 -> [_ w616 _]
            frame "Default", Default {
              n149 = case shown="Default" w561 {
                tunnel: w562 -> [w571 w598 w605 w614]
                tunnel: w560 -> [w570 w597 w607 w615]
                tunnel: [w568 w598 w599 w609] -> w559
                tunnel: [w565 w597 w606 w610] -> w558
                tunnel: [w569 _ w603 w612] -> w557
                tunnel: w556 -> [w563 _ _ _]
                frame "V", "v" {
                  # "Paste"
                  n150 = call "IE Read from Clipboard.vi"("error in"=w570, "Data in"=w571) -> ("error out"=w566:errorcluster, "Key Focus"=w569:bool, "Data out"=w567:T2, "Empty Clipboard string?"=w564:bool)  [unwired: 6 in]
                  n151 = case shown="True" w564 {
                    tunnel: [w574 w581] -> w568
                    tunnel: w567 -> [w573 w582]
                    tunnel: w566 -> [w572 w584]
                    tunnel: [w572 w578] -> w565
                    tunnel: w563 -> [_ w577]
                    frame False {
                      w576 = u32 111  # Invalid tool value
                      w575 = FALSE ("Support.CTRL Pressed")
                      n152 = Bundle By Name(cluster=w573, "Support.Shift pressed?"=w575, "Support.CTRL Pressed"=w575, "Support.Tool (old value)"=w576) -> (w574:T2)
                    }
                    frame True {
                      n153 = call "Empty Picture"() -> ("empty picture"=w585:picture)
                      n154 = call "Import_Clipboard.vi"("error in (no error)"=w584, "Picture in"=w585) -> ("error out"=w580:errorcluster, "Valid?"=w583:bool, "Picture"=w579:picture)  [unwired: 1 in, 6 out]
                      n155 = case shown="True" w583 {
                        tunnel: w582 -> [w587 w594]
                        tunnel: [w587 w590] -> w581
                        tunnel: w580 -> [w586 w595]
                        tunnel: w579 -> [_ w596]
                        tunnel: [w586 w589] -> w578
                        tunnel: w577 -> [_ w588]
                        frame False {
                        }
                        frame True {
                          n156 = call "Create new layer_LayerName_Picture.vi"("error in"=w595, "Layer name"=w588, "Picture"=w596, "Data in"=w594) -> ("error out"=w593:errorcluster, "Data out"=w592:T2)  [unwired: 6 in]
                          n157 = call "ViewLayer.vi"("Add to Undo?"=TRUE, "error in (no error)"=w593, "Data in"=w592) -> ("error out"=w589:errorcluster, "Data out"=w590:T2)  [unwired: 1 in, 6 out]
                        }
                      }
                    }
                  }
                }
                frame Default {
                }
                frame "C", "c" {
                  w602 = u32 111  # Invalid tool value
                  w601 = FALSE ("Support.CTRL Pressed")
                  n158 = call "IE Write to Clipboard.vi"("Is Cut?"=FALSE, "error in"=w607, "Data in"=w605) -> ("error out"=w606:errorcluster, "Key Focus"=w603:bool, "Data out"=w600:T2)  [unwired: 6 in]
                  n159 = Bundle By Name(cluster=w600, "Support.Shift pressed?"=w601, "Support.CTRL Pressed"=w601, "Support.Tool (old value)"=w602) -> (w599:T2)
                }
                frame "X", "x" {
                  n160 = call "IE Write to Clipboard.vi"("Is Cut?"=TRUE, "error in"=w615, "Data in"=w614) -> ("error out"=w611:errorcluster, "Key Focus"=w612:bool, "Data out"=w609:T2)  [unwired: 6 in]
                  n161 = Unbundle By Name(w609) -> ("Ref.Body Text"=w608:refnum<vi>)
                  n162 = call "Fire Body Text Change event.vi"("error in"=w611, "Ref.Body Text"=w608) -> ("error out"=w610:errorcluster)  [unwired: 9 in]
                }
              }
            }
            frame "Tool" {
              n163 = Compound Arithmetic op=AND(invert w623, w624) -> (w620:bool)
              n164 = case shown="\"V\", \"v\"" w619 {
                tunnel: w629 -> [w642 _ _ _]
                tunnel: w628 -> [w641 w694 w712 w721]
                tunnel: w627 -> [w638 w698 w714 w722]
                tunnel: [w637 w696 w713 w716] -> w626
                tunnel: [w635 w697 w711 w718] -> w625
                tunnel: w620 -> [w634 _ _ _]
                tunnel: w622 -> [w633 _ _ _]
                tunnel: w621 -> [w632 _ _ _]
                tunnel: [_ w693 w709 w717] -> w618
                tunnel: w617 -> [_ w695 _ _]
                tunnel: w616 -> [w631 _ _ _]
                frame Default {
                  n165 = call "IsAntsRectValid.vi"("AntsRect"=w631) -> ("Valid?"=w630:bool)  [unwired: 10 out]
                  n166 = property class="RadioBtnsControl (strict)"(reference=w642, error in=w641) -> (reference out=w636:refnum<vi>, error out=w639:errorcluster, "Value"=w640:T12)
                  n167 = case shown="\"Select\"" w640 {
                    selector: w640 -> [w649 w668 _]
                    tunnel: w639 -> [w647 w671 w691]
                    tunnel: w638 -> [w651 w673 w692]
                    tunnel: [w650 w672 w690] -> w637
                    tunnel: w634 -> [w648 _ _]
                    tunnel: w636 -> [w646 w669 _]
                    tunnel: [w645 w670 w691] -> w635
                    tunnel: w633 -> [w644 w667 w689]
                    tunnel: w632 -> [w643 w666 w688]
                    tunnel: w630 -> [_ w674 _]
                    frame "Pencil", Default {
                      n168 = case shown="False" w648 {
                        tunnel: w651 -> [w656 w660]
                        tunnel: [w654 w665] -> w650
                        tunnel: w649 -> [_ w664]
                        tunnel: w647 -> [w655 w659]
                        tunnel: w646 -> [_ w663]
                        tunnel: [w655 w662] -> w645
                        tunnel: w644 -> [_ w658]
                        tunnel: w643 -> [_ w657]
                        frame False {
                          w653 = u32 111  # Invalid tool value
                          w652 = FALSE ("Support.CTRL Pressed")
                          n169 = Bundle By Name(cluster=w656, "Support.Shift pressed?"=w652, "Support.CTRL Pressed"=w652, "Support.Tool (old value)"=w653) -> (w654:T2)
                        }
                        frame True {
                          n170 = property class="RadioBtnsControl (strict)"(reference=w663, error in=w659, "Val(Sgnl)"=T12."Dropper" ("Value (Signaling)")) -> (error out=w662:errorcluster)  [unwired: 1 out]
                          n171 = Bundle By Name(cluster=w660, "Support.Tool (old value)"=w664, "Support.Shift pressed?"=w658, "Support.CTRL Pressed"=w657) -> (w665:T2)
                        }
                      }
                    }
                    frame "Select" {
                      n172 = case shown="True" w674 {
                        tunnel: w673 -> [w679 w687]
                        tunnel: [w678 w685] -> w672
                        tunnel: w671 -> [w682 w686]
                        tunnel: [w681 w686] -> w670
                        tunnel: w669 -> [w680 _]
                        tunnel: w668 -> [w677 _]
                        tunnel: w667 -> [w676 _]
                        tunnel: w666 -> [w675 _]
                        frame False {
                          n173 = Bundle By Name(cluster=w679, "Support.Tool (old value)"=w677, "Support.Shift pressed?"=w676, "Support.CTRL Pressed"=w675) -> (w678:T2)
                          n174 = property class="RadioBtnsControl (strict)"(reference=w680, error in=w682, "Val(Sgnl)"=T12."Dropper" ("Value (Signaling)")) -> (error out=w681:errorcluster)  [unwired: 1 out]
                        }
                        frame True {
                          w684 = u32 111  # Invalid tool value
                          n175 = Bundle By Name(cluster=w687, "Support.Tool (old value)"=w684) -> (w685:T2)
                        }
                      }
                    }
                    frame "Dropper" {
                      n176 = Bundle By Name(cluster=w692, "Support.Shift pressed?"=w689, "Support.CTRL Pressed"=w688) -> (w690:T2)
                    }
                  }
                }
                frame "V", "v" {
                  n177 = call "IE Read from Clipboard.vi"("error in"=w694, "Data in"=w698) -> ("error out"=w700:errorcluster, "Key Focus"=w693:bool, "Data out"=w701:T2, "Empty Clipboard string?"=w699:bool)  [unwired: 6 in]
                  n178 = case shown="False" w699 {
                    tunnel: [w704 w707] -> w696
                    tunnel: w701 -> [w703 w707]
                    tunnel: w700 -> [w702 w708]
                    tunnel: [w702 w708] -> w697
                    tunnel: w695 -> [_ _]
                    frame False {
                      w706 = u32 111  # Invalid tool value
                      w705 = FALSE ("Support.CTRL Pressed")
                      n179 = Bundle By Name(cluster=w703, "Support.Shift pressed?"=w705, "Support.CTRL Pressed"=w705, "Support.Tool (old value)"=w706) -> (w704:T2)
                    }
                    frame True {
                    }
                  }
                }
                frame "C", "c" {
                  n180 = call "IE Write to Clipboard.vi"("Is Cut?"=FALSE, "error in"=w712, "Data in"=w714) -> ("error out"=w711:errorcluster, "Key Focus"=w709:bool, "Data out"=w713:T2)  [unwired: 6 in]
                }
                frame "X", "x" {
                  n181 = call "IE Write to Clipboard.vi"("Is Cut?"=TRUE, "error in"=w721, "Data in"=w722) -> ("error out"=w719:errorcluster, "Key Focus"=w717:bool, "Data out"=w716:T2)  [unwired: 6 in]
                  n182 = Unbundle By Name(w716) -> ("Ref.Body Text"=w715:refnum<vi>)
                  n183 = call "Fire Body Text Change event.vi"("error in"=w719, "Ref.Body Text"=w715) -> ("error out"=w718:errorcluster)  [unwired: 9 in]
                }
              }
            }
            frame "Move Selection" {
              n184 = case shown="\"Z\", \"z\"" w729 {
                tunnel: w726 -> [w732 w739 w751]
                tunnel: w731 -> [w733 w738 w752]
                tunnel: [w733 w737 w749] -> w730
                tunnel: w728 -> [_ w736 _]
                tunnel: [_ w735 _] -> w727
                tunnel: [w732 w734 w750] -> w725
                tunnel: w724 -> [_ _ _]
                tunnel: w723 -> [_ _ _]
                frame Default {
                }
                frame "Z", "z" {
                  n185 = case shown="False" w736 {
                    tunnel: w739 -> [w743 w746]
                    tunnel: w738 -> [w745 w748]
                    tunnel: [w744 w748] -> w737
                    tunnel: [TRUE TRUE] -> w735
                    tunnel: [w742 w746] -> w734
                    frame False {
                      n186 = call "Escape.vi"("Reset cursor (T)"=FALSE, "error in"=w743, "Data in"=w745) -> ("error out"=w742:errorcluster, "Data out"=w744:T2)  [unwired: 7 out]
                    }
                    frame True {
                    }
                  }
                }
                frame "V", "v" {
                  n187 = call "Finalize Movement.vi"("error in (no error)"=w751, "Data in"=w752) -> ("error out"=w750:errorcluster, "Data out"=w749:T2)  [unwired: 2 in, 6 out]
                }
              }
            }
          }
          n188 = Or(x=w537, y=w543) -> (x .or. y?=w538:bool)
        }
      }
    }
    frame Error {
    }
  }
  "error out" <- w9
  "Discard?" <- w5
  "Data out" <- w3
